vi "Compare_Checksums.vi"(8 "error in (no error)":errorcluster, 10 "build object":T1, 11 "PreviewCache":refnum<class "PreviewCache.lvclass">) -> (0 "error out":errorcluster, 2 "valid?":bool, 3 "PreviewCache out":refnum<class "PreviewCache.lvclass">)   [LabVIEW 2020, in "PreviewCache.lvclass"]
uses:
  <vilib>/AppBuilder/AB_Classes/PreviewCache/PreviewCache.lvclass
  <resource>/Framework/Providers/API/ItemRef.ctl
  <vilib>/AppBuilder/AB_Classes/PreviewCache/PreviewCache.lvclass/PreviewCache.ctl
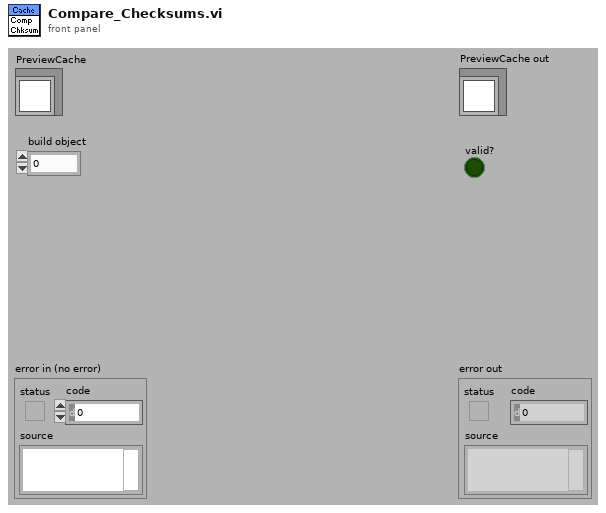
[diagram p1: front panel]
types:
  T1 = typedef "ItemRef.ctl" = u64
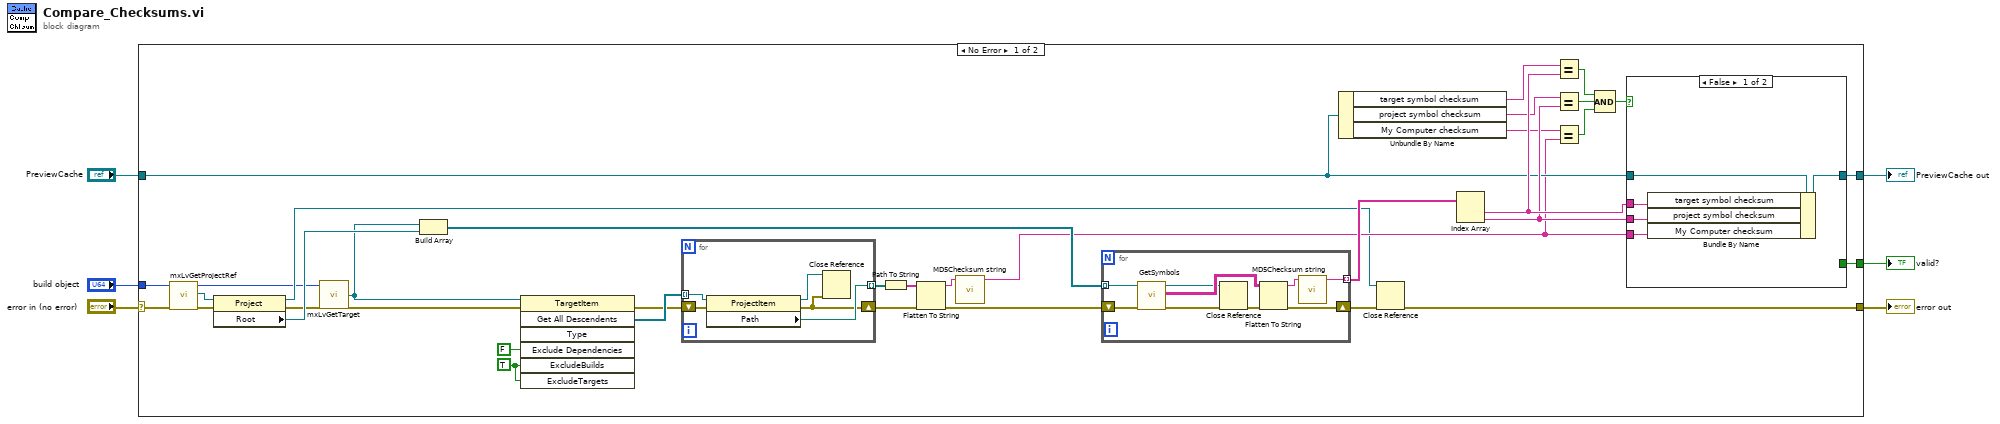
[diagram p0: block diagram]
diagram:
  n1 = case shown="No Error" "error in (no error)" {
    selector: "error in (no error)" -> [w23 w64]
    tunnel: [w42 w64] -> w6
    tunnel: [w25 _] -> w5
    tunnel: [w41 _] -> w4
    tunnel: "PreviewCache" -> [w24 _]
    tunnel: "build object" -> [w22 _]
    frame No Error {
      w15 = TRUE ("ExcludeTargets")
      n2 = call <resource>:"mxLvGetProjectRef.vi"("error in"=w23, "Item"=w22) -> ("error out"=w37:errorcluster, "Project Refnum"=w40:refnum<vi>, "Item"=w7:T1)  [unwired: 7 in]
      n3 = property class="Project"(reference=w40, error in=w37) -> (reference out=w11:refnum<vi>, error out=w9:errorcluster, "Root"=w39:refnum<vi>)
      n4 = call <resource>:"mxLvGetTarget.vi"("Item"=w7, "error in"=w9) -> ("Target"=w10:refnum<vi>, "error out"=w8:errorcluster)  [unwired: 1 out]
      n5 = Build Array(w10, w39) -> (w38:refnum<vi>[])
      n6 = invoke class="TargetItem" method="Get All Descendents"(reference=w10, error in=w8, "Exclude Dependencies"=FALSE ("ExcludeDependencies"), "ExcludeBuilds"=w15, "ExcludeTargets"=w15) -> (error out=w17:errorcluster, "All Descendents"=w21:refnum<vi>[])  [unwired: 2 in, 5 out]
      n7 = for {
        tunnel: w21 -> [w47] mode=indexing
        tunnel: [w46] -> w20 mode=indexing
        shift-right: [w43] -> w16
        shift-left: w17 -> [w44]
        n8 = property class="ProjectItem"(reference=w47, error in=w44) -> (reference out=w45:refnum<vi>, error out=w43:errorcluster, "Path"=w46:path)
        n9 = Close Reference(reference=w45, error in (no error)=w43) -> ()  [unwired: 1 out]
      }
      n10 = Path To String(path=w20) -> (string=w18:string[])
      n11 = Flatten To String(anything=w18, error in (no error)=w16) -> (data string=w19:string, error out=w14:errorcluster)  [unwired: 3 out]
      n12 = call <vilib>:"MD5Checksum string.vi"("Message String"=w19) -> ("MD5 message-digest"=w13:string)  [unwired: 10 out]
      n13 = for {
        tunnel: w38 -> [w55] mode=indexing
        tunnel: [w51] -> w34 mode=indexing
        shift-right: [w48] -> w36
        shift-left: w14 -> [w49]
        n14 = call <resource>:"GetSymbols.vi"("error in"=w49, "Project Item"=w55) -> ("error out"=w53:errorcluster, "Symbol Value Pairs"=w56:string[][], "Project Item"=w50:refnum<vi>)  [unwired: 6 in, 1 out]
        n15 = Close Reference(reference=w50, error in (no error)=w53) -> (error out=w52:errorcluster)
        n16 = Flatten To String(anything=w56, error in (no error)=w52) -> (data string=w54:string, error out=w48:errorcluster)  [unwired: 3 out]
        n17 = call <vilib>:"MD5Checksum string.vi"("Message String"=w54) -> ("MD5 message-digest"=w51:string)  [unwired: 10 out]
      }
      n18 = Unbundle By Name(w24) -> ("target symbol checksum"=w33:string, "project symbol checksum"=w31:string, "My Computer checksum"=w29:string)
      n19 = Close Reference(reference=w11, error in (no error)=w36) -> (error out=w42:errorcluster)
      n20 = Index Array(array=w34) -> (element #1=w32:string, element #2=w30:string)  [unwired: 2 in]
      n21 = Equal?(x=w33, y=w32) -> (x = y?=w28:bool)
      n22 = Equal?(x=w31, y=w30) -> (x = y?=w27:bool)
      n23 = Equal?(x=w29, y=w13) -> (x = y?=w26:bool)
      n24 = Compound Arithmetic op=AND(w28, w27, w26) -> (w35:bool)
      n25 = case shown="False" w35 {
        selector: w35 -> [_ w63]
        tunnel: w32 -> [w61 _]
        tunnel: w30 -> [w60 _]
        tunnel: w13 -> [w59 _]
        tunnel: [_ w63] -> w41
        tunnel: w24 -> [w58 w62]
        tunnel: [w57 w62] -> w25
        frame False {
          n26 = Bundle By Name(cluster=w58, "target symbol checksum"=w61, "project symbol checksum"=w60, "My Computer checksum"=w59) -> (w57:refnum<class "PreviewCache.lvclass">)
        }
        frame True {
        }
      }
    }
    frame Error {
    }
  }
  "error out" <- w6
  "PreviewCache out" <- w5
  "valid?" <- w4
